vi "DetectPressureAnomalies.vi"(3 "Pressure Loss Threshold (psi/min)":dbl=-5.0, 4 "Compressor Running":bool, 5 "Pressure (psi)":dbl(slide) scale=0.0..120.0) -> (0 "Pressure Change (psi/min)":dbl, 1 "Pressure Leak":bool, 2 "Pressure Vent":bool)   [LabVIEW 2020]
doc: "This VI can detect both rapid pressure venting events and slow pressure leak conditions."
uses:
  <vilib>/Rock Robotics/WPI/DriverStation/WPI_DriverStationRobotMode2.ctl
  driverdata.vi
  <vilib>/Analysis/NI_AALPro.lvlib
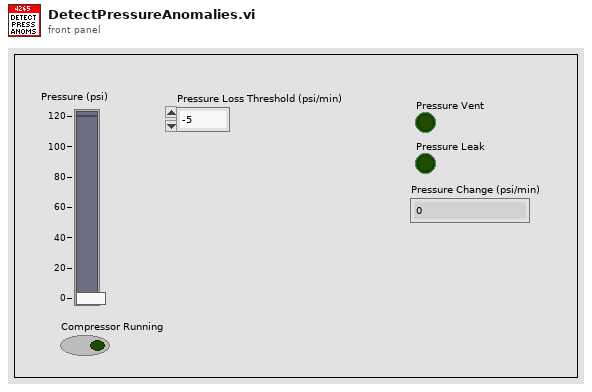
[diagram p1: front panel]
types:
  T1 = typedef "WPI_DriverStationRobotMode2.ctl" = enum16{"Autonomous Disabled", "Autonomous Enabled", "Teleop Disabled", "Teleop Enabled", "Disconnected", "Finish", "Test Disabled", "Test Enabled", "Emergency Stopped"}
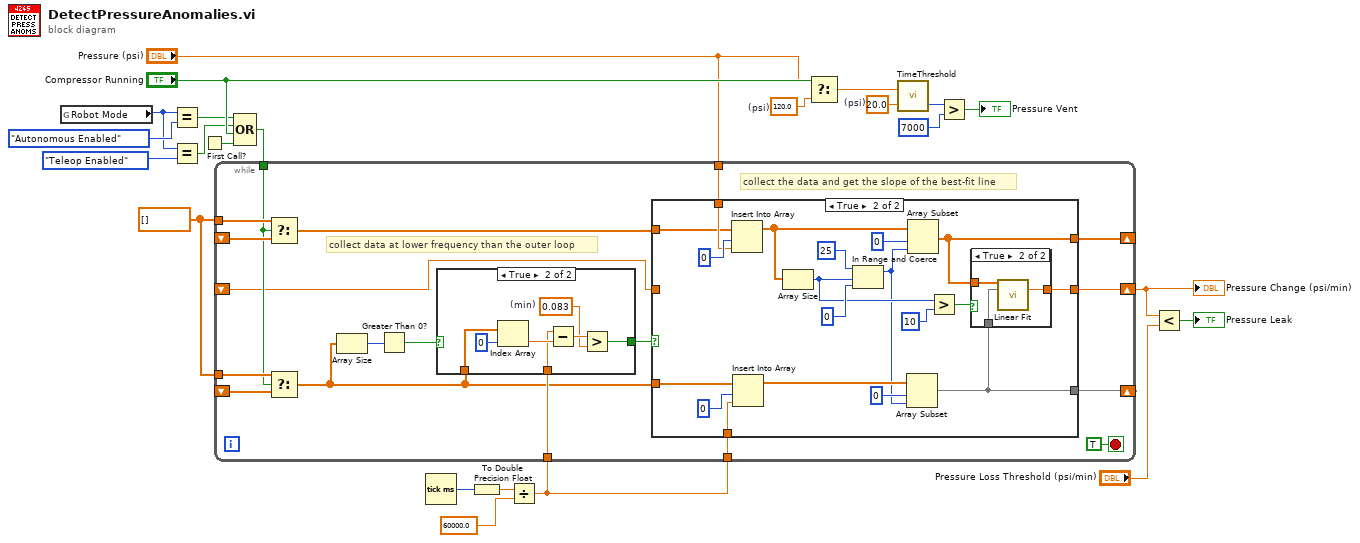
[diagram p0: block diagram]
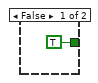
[diagram p2: hidden frame]
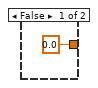
[diagram p4: hidden frame]
diagram:
  w11 = dbl[] [] ("array")
  w22 = 120.0  # (psi)
  w23 = 20.0  # (psi)
  n1 = global read "driverdata.vi" "Robot Mode"() -> (w3:T1)
  n2 = Equal?(x=w3, y=WPI_DriverStationRobotMode2."Autonomous Enabled" ("Robot Mode")) -> (x = y?=w4:bool)
  n3 = Equal?(x=w3, y=WPI_DriverStationRobotMode2."Teleop Enabled") -> (x = y?=w1:bool)
  n4 = First Call?() -> (First Call?: T/F=w17:bool)
  n5 = Compound Arithmetic op=OR(w4, w1, "Compressor Running", w17) -> (w15:bool)
  n6 = Tick Count (ms)() -> (millisecond timer value=w14:u32)
  n7 = To Double Precision Float(number=w14) -> (double precision float=w13:dbl)
  n8 = Divide(x=w13, y=60000.0) -> (x/y=w7:dbl)
  n9 = while {
    tunnel: "Pressure (psi)" -> [w40]
    shift-right: [w37] -> _
    shift-left: _ -> [w39]
    tunnel: w11 -> [w38]
    tunnel: w15 -> [w32]
    tunnel: w7 -> [w34]
    tunnel: w11 -> [w33]
    shift-right: [w31] -> _
    shift-left: _ -> [w30]
    tunnel: w7 -> [w29]
    shift-right: [w36] -> w10
    shift-left: _ -> [w24]
    stop <- TRUE stop-if-true
    # "collect the data and get the slope of the best-fit line"
    # "collect data at lower frequency than the outer loop"
    n10 = Select(t=w38, s=w32, f=w39) -> (s? t:f=w35:dbl[])
    n11 = Select(t=w33, s=w32, f=w30) -> (s? t:f=w27:dbl[])
    n12 = Array Size(array=w27) -> (size(s)=w26:i32)
    n13 = Greater Than 0?(x=w26) -> (x > 0?=w25:bool)
    n14 = case shown="True" w25 {
      tunnel: w29 -> [_ w47]
      tunnel: [TRUE w44] -> w28
      tunnel: w27 -> [_ w43]
      frame False {
      }
      frame True {
        w45 = 0.083  # (min)
        n15 = Index Array(array=w43, index=0) -> (element=w48:dbl)
        n16 = Subtract(x=w47, y=w48) -> (x-y=w46:dbl)
        n17 = Greater?(x=w46, y=w45) -> (0:w44:bool)
      }
    }
    n18 = case shown="True" w28 {
      tunnel: w40 -> [_ w70]
      tunnel: [w52 w65] -> w37
      tunnel: [w50 w61] -> w36
      tunnel: w35 -> [w52 w59]
      tunnel: w34 -> [_ w58]
      tunnel: [w51 w54] -> w31
      tunnel: w27 -> [w51 w53]
      tunnel: w24 -> [w50 _]
      frame False {
      }
      frame True {
        n19 = Insert Into Array(array=w59, index=0, new element=w70) -> (w68:dbl[])
        n20 = Insert Into Array(array=w53, index=0, new element=w58) -> (w56:dbl[])
        n21 = Array Size(array=w68) -> (size(s)=w63:i32)
        n22 = In Range and Coerce(upper limit=25, x=w63, lower limit=0) -> (coerced(x)=w55:i32)  [unwired: 1 out]
        n23 = Array Subset(array=w56, index=0, length=w55) -> (w54:dbl[])
        n24 = Array Subset(array=w68, index=0, length=w55) -> (w65:dbl[])
        n25 = Greater?(x=w63, y=10) -> (0:w64:bool)
        n26 = case shown="True" w64 {
          tunnel: w65 -> [_ w75]
          tunnel: [0.0 ("slope") w74] -> w61
          tunnel: w54 -> [_ w73]
          frame False {
          }
          frame True {
            n27 = call <vilib>:"Linear Fit.vi"("Y"=w75, "X"=w73) -> ("slope"=w74:dbl)  [unwired: 9 in, 4 out]
          }
        }
      }
    }
  }
  "Pressure Change (psi/min)" <- w10
  n28 = Select(t="Pressure (psi)", s="Compressor Running", f=w22) -> (s? t:f=w21:dbl)
  n29 = call "TimeThreshold.vi"("Threshold"=w23, "Current Value"=w21) -> ("Time Below Threshold (ms)"=w20:u32)  [unwired: 1 out]
  n30 = Greater?(x=w20, y=u32 7000) -> (0:→"Pressure Vent":bool)
  n31 = Less?(x=w10, y="Pressure Loss Threshold (psi/min)") -> (x < y?=→"Pressure Leak":bool)
